vi "Read Status.vi"(8 "error in (no error)":errorcluster, 11 "IgusMotorDrive in":refnum<class "IgusMotorDrive.lvclass">) -> (0 "error out":errorcluster, 2 "Status":T1, 3 "IgusMotorDrive out":refnum<class "IgusMotorDrive.lvclass">)   [LabVIEW 2016, in "IgusMotorDrive.lvclass"]
uses:
  IgusMotorDrive.lvclass
  motor-drive/MotorDrive.lvclass
  motor-drive/Globals/Status--cluster.ctl
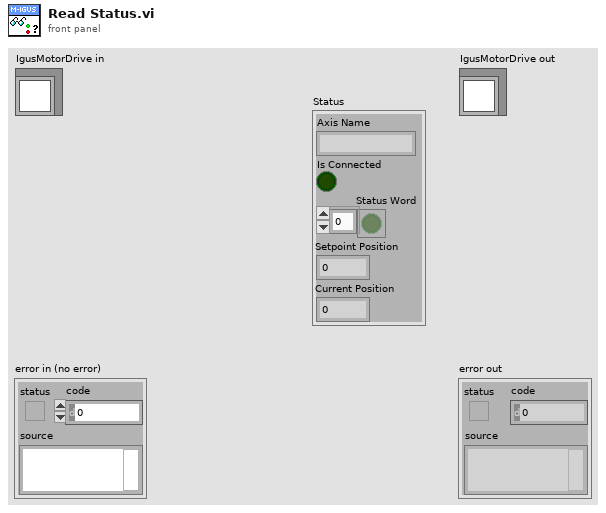
[diagram p1: front panel]
types:
  T1 = typedef "MotorDrive.lvclass/Status--cluster.ctl" = cluster{"Axis Name":string, "Is Connected":bool, "Status Word":bool[], "Setpoint Position":dbl, "Current Position":dbl}
  T2 = typedef "IgusMotorDrive.lvclass/Statusword--cluster.ctl" = cluster{"Ready to Switch On":bool, "Switched On":bool, "Operation Enabled":bool, "Fault":bool, "Voltage Enabled":bool, "Quick Stop":bool, "Switch On Disabled":bool, "Warning":bool, "8 Manufacturer Specific":bool, "Remote":bool, "Home Successful/Target Reached":bool, "Internal Limit Active":bool, "12 MS (0:Homing/1:Homed)":bool, "13 MS":bool, "14 Manufacturer Specific":bool, "15 Manufacturer Specific":bool}
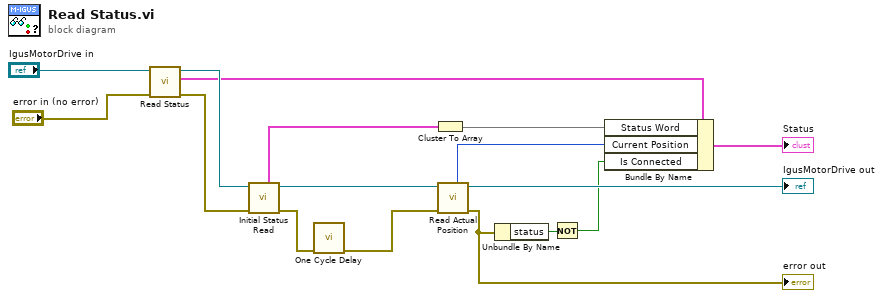
[diagram p0: block diagram]
diagram:
  n1 = call-parent "Read Status.vi"("error in (no error)"="error in (no error)", "MotorDrive in"="IgusMotorDrive in") -> ("error out"=w13:errorcluster, "Status"=w8:T1, "MotorDrive out"=w11:refnum<class "IgusMotorDrive.lvclass">)  [unwired: 7 in]
  n2 = call "Initial Status Read.vi"("error in (no error)"=w13, "IgusMotorDrive in"=w11) -> ("error out"=w12:errorcluster, "IgusMotorDrive out"=w10:refnum<class "IgusMotorDrive.lvclass">, "Statusword out"=w5:T2)  [unwired: 4 in, 3 out]
  n3 = call "One Cycle Delay.vi"("error in (no error)"=w12) -> ("error out"=w14:errorcluster)  [unwired: 10 in]
  n4 = Cluster To Array(cluster=w5) -> (array=w6:bool[])
  n5 = call "Read Actual Position.vi"("error in (no error)"=w14, "IgusMotorDrive in"=w10) -> ("error out"=w3:errorcluster, "IgusMotorDrive out"=→"IgusMotorDrive out":refnum<class "IgusMotorDrive.lvclass">, "Position"=w7:i32)  [unwired: 5 in, 2 out]
  "error out" <- w3
  n6 = Unbundle By Name(w3) -> ("status"=w2:bool)
  n7 = Not(x=w2) -> (.not. x?=w1:bool)
  n8 = Bundle By Name(cluster=w8, "Status Word"=w6, "Current Position"=w7, "Is Connected"=w1) -> (→"Status":T1)
